vi "all-signals_counter-error.vi"() -> ()   [LabVIEW 2018]
uses:
  <vilib>/Analysis/baseanly.llb/Mean (DBL).vi
  <vilib>/Analysis/NI_AALBase.lvlib
panel:
  in  "Tab Control":T1(tab)
  in  "stop I,U,M_brems (F)":bool caption="M_brems, elektr. P stop (F)"
  in  "stop  counter (F)":bool caption="counter stop (F)"
  in  "stop clear charts":bool
  in  "stop driving torque":bool
  in  "Messzeit in ms":u32=100 min=10 max=1000 step=10
  in  "Clear Charts":bool
  out "driving torque and counter":dynamicdata(graph)
  out "M_mech/N_motor":cluster{"Y":dbl[], "Y":dbl[]}[](graph)
  out "driving torque selected":dbl(graph)
  out "Motordrehzahl":dynamicdata(graph)
  out "Driving Torque gemittelt":dbl(graph)
  out "RPM and dn":dynamicdata(graph)
  out "Geschwindigkeit":dynamicdata(graph)
  out "Elektrische Leistung":waveform(dbl)(graph)
  out "RPM":dbl
  out "Bremsmoment":dynamicdata(graph)
  out "angular acc":dynamicdata(graph)
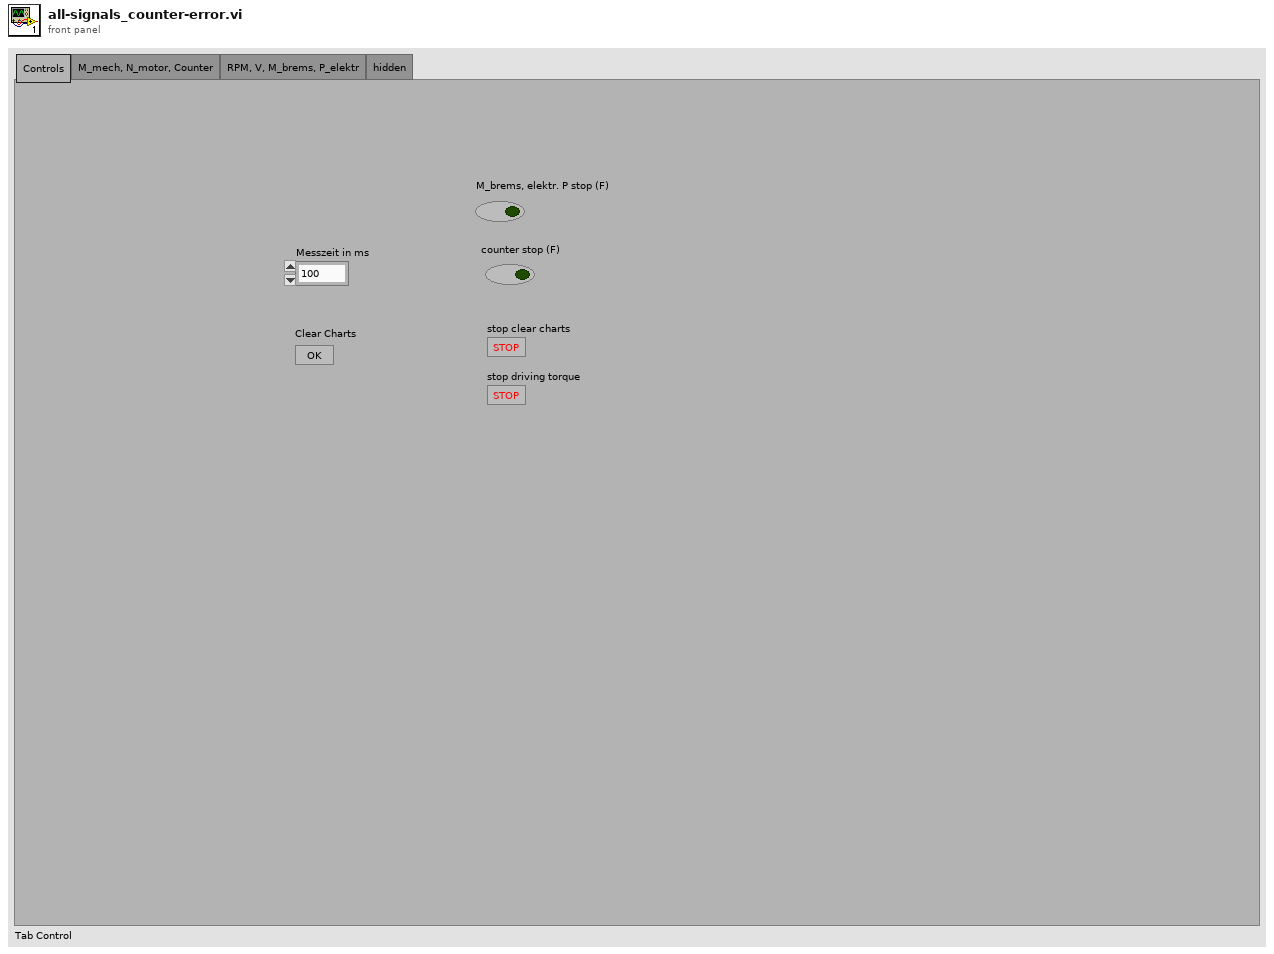
[diagram p1: front panel]
types:
  T1 = enum32{"Controls", "M_mech, N_motor, Counter", "RPM, V, M_brems, P_elektr", "hidden"}
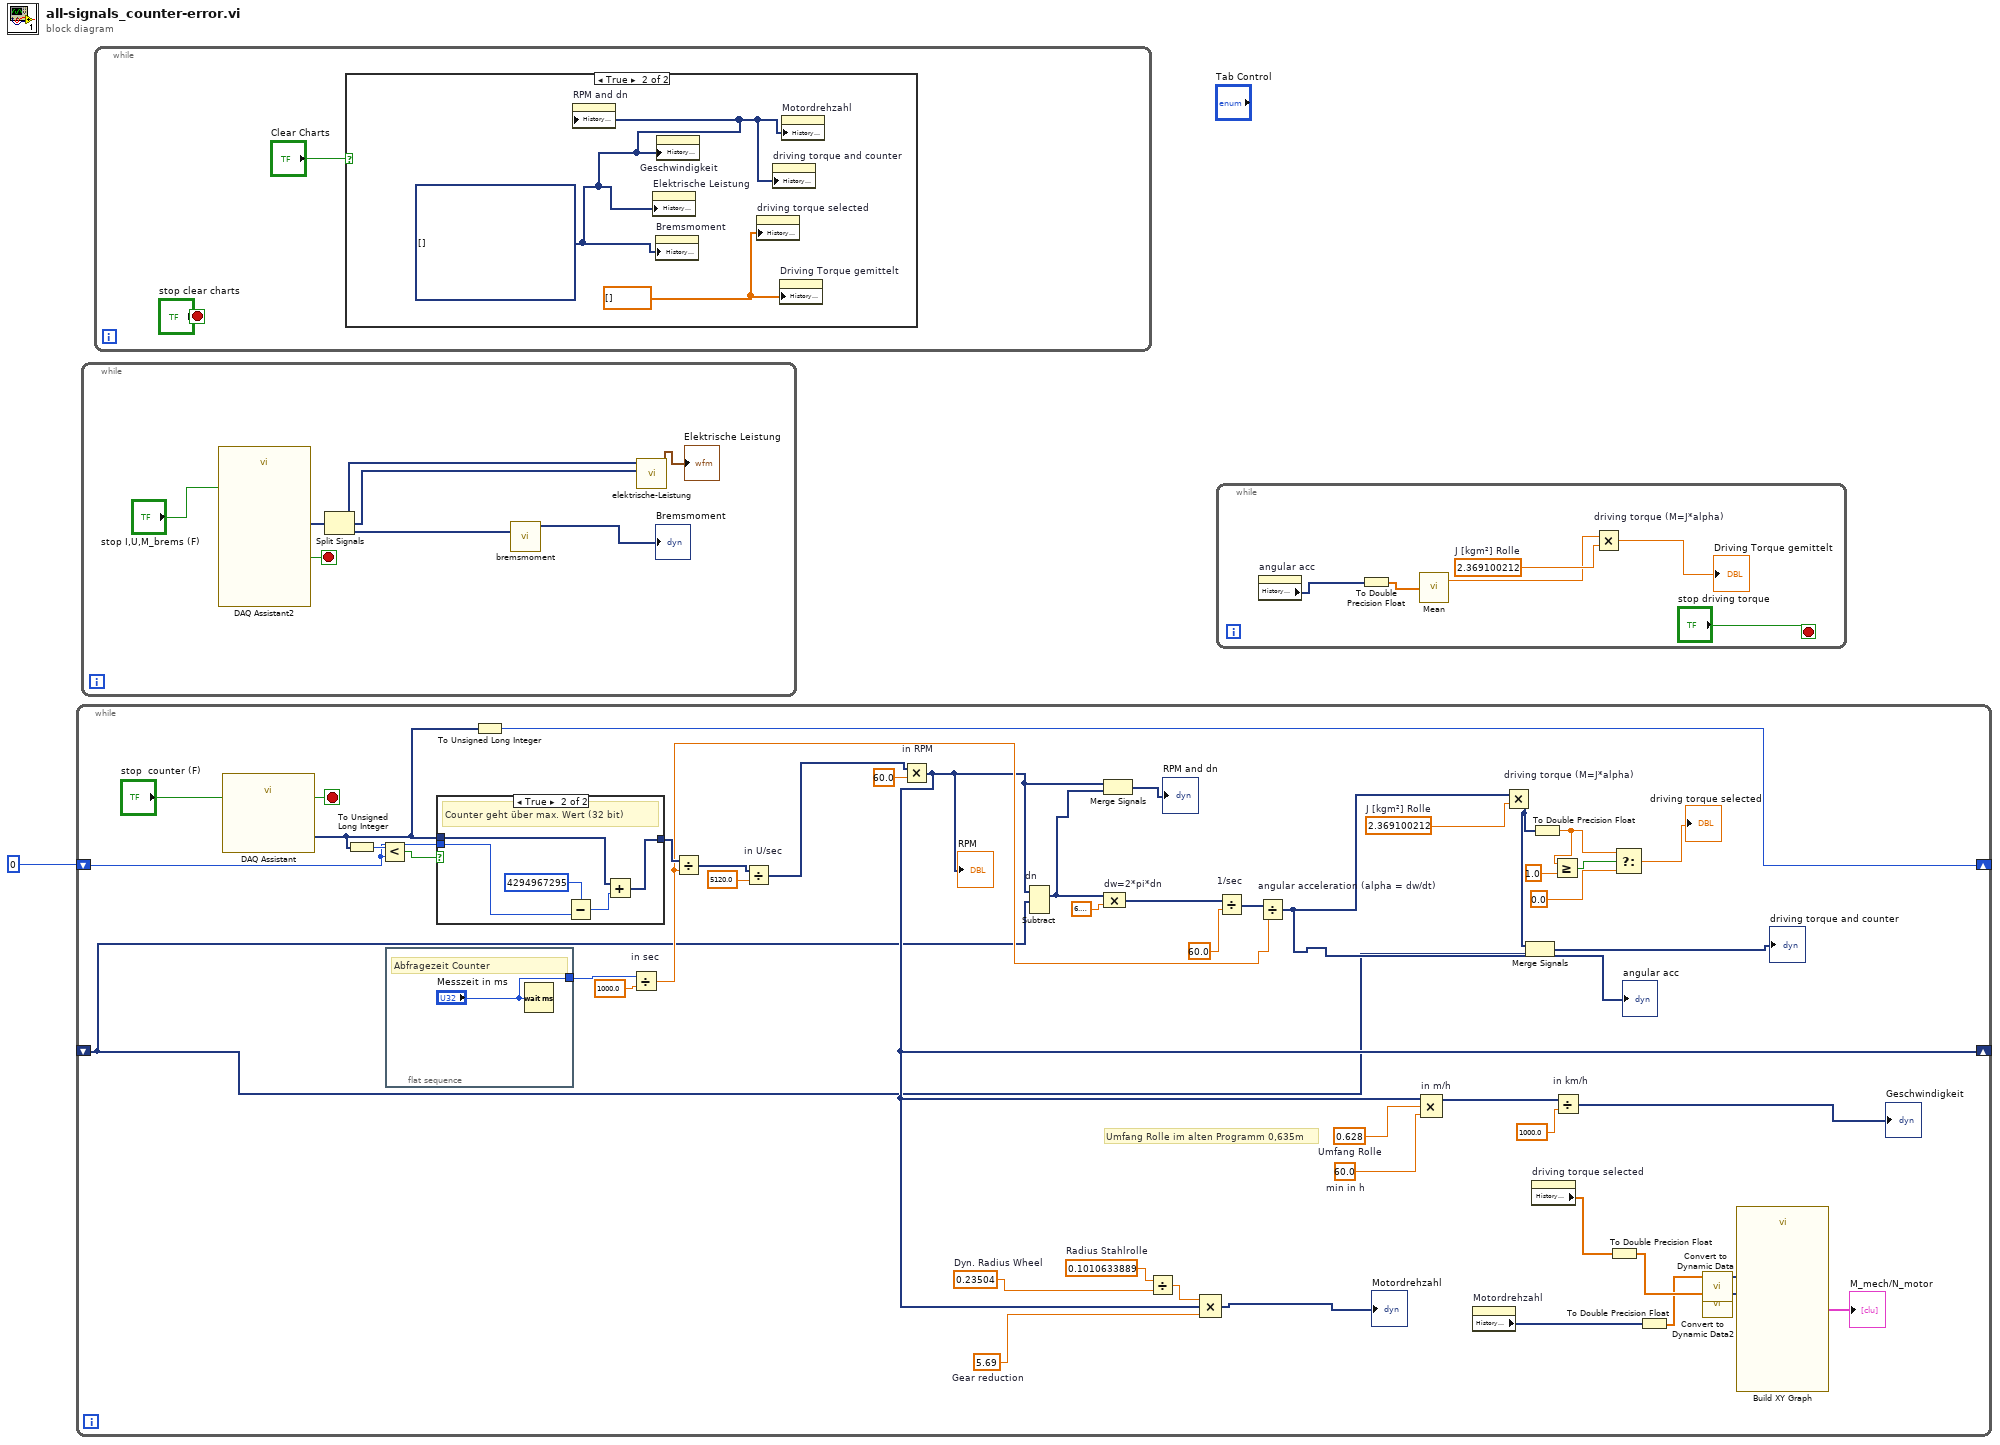
[diagram p0: block diagram]
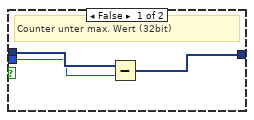
[diagram p2: hidden frame]
diagram:
  n1 = while {
    shift-right: [w48] -> _
    shift-left: u32 0 -> [w27]
    shift-right: [w22] -> _
    shift-left: _ -> [w2]
    stop <- w46 stop-if-true
    w19 = 2.369100212  # J [kgm²] Rolle
    w20 = 5.69  # Gear reduction
    w21 = 0.23504  # Dyn. Radius Wheel
    w24 = 0.1010633889  # Radius Stahlrolle
    w33 = 60.0  # min in h
    w32 = 0.628  # Umfang Rolle
    # "Umfang Rolle im alten Programm 0,635m"
    n2 = call "DAQ Assistant"("stop (F)"="stop  counter (F)") -> ("data"=w28:dynamicdata, "stopped"=w46:bool)  [unwired: 15 in, 2 out]
    n3 = To Unsigned Long Integer(number=w28) -> (unsigned 32bit integer=w47:u32)
    n4 = Less?(x=w47, y=w27) -> (x < y?=w50:bool)
    n5 = flat-sequence {
      tunnel: ["Messzeit in ms"] -> w45
      frame #0 {
        # "Abfragezeit Counter"
        n6 = Wait (ms)(milliseconds to wait="Messzeit in ms") -> ()  [unwired: 1 out]
      }
    }
    n7 = case shown="True" w50 {
      tunnel: w28 -> [w54 w56]
      tunnel: w27 -> [w53 w58]
      tunnel: [w52 w55] -> w43
      frame False {
        # "Counter unter max. Wert (32bit)"
        n8 = Subtract(x=w54, y=w53) -> (x-y=w52:dynamicdata)
      }
      frame True {
        # "Counter geht über max. Wert (32 bit)"
        n9 = Subtract(x=u32 4294967295, y=w58) -> (x-y=w57:u32)
        n10 = Add(x=w56, y=w57) -> (x+y=w55:dynamicdata)
      }
    }
    n11 = To Unsigned Long Integer(number=w28) -> (unsigned 32bit integer=w48:u32)
    n12 = Divide "in sec"(x=w45, y=1000.0) -> (x/y=w36:dbl)
    n13 = Divide(x=w43, y=w36) -> (x/y=w42:dynamicdata)
    n14 = Divide "in U/sec"(x=w42, y=5120.0) -> (x/y=w30:dynamicdata)
    n15 = Multiply "in RPM"(x=w30, y=60.0) -> (x*y=w22:dynamicdata)
    "RPM" <- w22
    n16 = Subtract "dn"(1:w2, 2:w22) -> (0:w25:dynamicdata)  [unwired: 1 in, 1 out]
    n17 = Merge Signals(w22, w25) -> (→"RPM and dn":dynamicdata)
    n18 = Compound Arithmetic op=MULTIPLY "dw=2*pi*dn"(w25, 6.283185307179586) -> (w39:dynamicdata)
    n19 = Divide(x=w24, y=w21) -> (x/y=w23:dbl)
    n20 = Compound Arithmetic op=MULTIPLY(w23, w22, w20) -> (→"Motordrehzahl":dynamicdata)
    n21 = Divide "1/sec"(x=w39, y=60.0) -> (x/y=w37:dynamicdata)
    n22 = Divide "angular acceleration (alpha = dw/dt)"(x=w37, y=w36) -> (x/y=w4:dynamicdata)
    "angular acc" <- w4
    n23 = Compound Arithmetic op=MULTIPLY "in m/h"(w22, w32, w33) -> (w34:dynamicdata)
    n24 = property on="Motordrehzahl" class="WFChart (strict)"() -> ("History Data"=w12:dynamicdata[])  [unwired: 2 in, 2 out]
    n25 = Multiply "driving torque (M=J*alpha)"(x=w4, y=w19) -> (x*y=w10:dynamicdata)
    n26 = Merge Signals(w10, w2) -> (→"driving torque and counter":dynamicdata)
    n27 = property on="driving torque selected" class="WFChart (strict)"() -> ("History Data"=w18:dbl[])  [unwired: 2 in, 2 out]
    n28 = To Double Precision Float(number=w10) -> (double precision float=w9:dbl)
    n29 = Greater Or Equal?(x=w9, y=1.0) -> (x >= y?=w7:bool)
    n30 = Divide "in km/h"(x=w34, y=1000.0) -> (x/y=→"Geschwindigkeit":dynamicdata)
    n31 = To Double Precision Float(number=w18) -> (double precision float=w17:dbl[])
    n32 = Select(t=w9, s=w7, f=0.0) -> (s? t:f=→"driving torque selected":dbl)
    n33 = To Double Precision Float(number=w12) -> (double precision float=w14:dbl[])
    n34 = call "Convert to Dynamic Data"("Array"=w14) -> ("Dynamic Data Type"=w15:dynamicdata)  [unwired: 3 in]
    n35 = call "Convert to Dynamic Data2"("Array"=w17) -> ("Dynamic Data Type"=w16:dynamicdata)  [unwired: 3 in]
    n36 = call "Build XY Graph"("Y Input"=w16, "X Input"=w15) -> ("XY Graph"=→"M_mech/N_motor":cluster{"X":dbl[], "Y":dbl[]}[])  [unwired: 8 in, 1 out]
  }
  n37 = while {
    stop <- w62 stop-if-true
    n38 = call "DAQ Assistant2"("stop (F)"="stop I,U,M_brems (F)") -> ("data"=w63:dynamicdata, "stopped"=w62:bool)  [unwired: 15 in, 2 out]
    n39 = Split Signals(w63) -> (w67:dynamicdata, w66:dynamicdata, w65:dynamicdata)  [unwired: 3 in]
    n40 = call "bremsmoment.vi"("Dynamic Data in"=w65) -> ("Dynamic Data out"=→"Bremsmoment":dynamicdata)  [unwired: 10 in]
    n41 = call "elektrische-Leistung.vi"("Dynamic Data"=w66, "Dynamic Data 2"=w67) -> ("Elektrische Leistung"=→"Elektrische Leistung":waveform(dbl))  [unwired: 9 in]
  }
  n42 = while {
    stop <- "stop clear charts" stop-if-true
    n43 = case shown="True" "Clear Charts" {
      frame False {
      }
      frame True {
        w71 = dbl[] [] ("History Data")
        w70 = dynamicdata[] [] ("History Data")
        n44 = property on="RPM and dn" class="WFChart (strict)"("History Data"=w70) -> ()  [unwired: 2 in, 2 out]
        n45 = property on="Elektrische Leistung" class="WFChart (strict)"("History Data"=w70) -> ()  [unwired: 2 in, 2 out]
        n46 = property on="Bremsmoment" class="WFChart (strict)"("History Data"=w70) -> ()  [unwired: 2 in, 2 out]
        n47 = property on="Geschwindigkeit" class="WFChart (strict)"("History Data"=w70) -> ()  [unwired: 2 in, 2 out]
        n48 = property on="driving torque selected" class="WFChart (strict)"("History Data"=w71) -> ()  [unwired: 2 in, 2 out]
        n49 = property on="driving torque and counter" class="WFChart (strict)"("History Data"=w70) -> ()  [unwired: 2 in, 2 out]
        n50 = property on="Driving Torque gemittelt" class="WFChart (strict)"("History Data"=w71) -> ()  [unwired: 2 in, 2 out]
        n51 = property on="Motordrehzahl" class="WFChart (strict)"("History Data"=w70) -> ()  [unwired: 2 in, 2 out]
      }
    }
  }
  n52 = while {
    stop <- "stop driving torque" stop-if-true
    w76 = 2.369100212  # J [kgm²] Rolle
    n53 = property on="angular acc" class="WFChart (strict)"() -> ("History Data"=w72:dynamicdata[])  [unwired: 2 in, 2 out]
    n54 = To Double Precision Float(number=w72) -> (double precision float=w77:dbl[])
    n55 = call-poly <vilib>:"Mean.vi"("X"=w77) -> ("mean"=w74:dbl)  [unwired: 1 out]
    n56 = Multiply "driving torque (M=J*alpha)"(x=w74, y=w76) -> (x*y=→"Driving Torque gemittelt":dbl)
  }
